vi "Current Loop 9505 (FPGA) - bef combining sample current loops.vi"() -> ()   [LabVIEW 2011]
uses:
  <vilib>/LabVIEW Targets/FPGA/cRIO/cRIO-9505/controls.llb/_nicrio_cRIO-9505_DriveStatus.ctl
  <vilib>/Platform/TimedLoop/XDataNode/timing_clust.ctl
  <vilib>/Platform/TimedLoop/XDataNode/nitl_modes.ctl
  <vilib>/Platform/TimedLoop/XDataNode/wakeup.ctl
  <vilib>/LabVIEW Targets/FPGA/cRIO/cRIO-9505/controls.llb/_nicrio_cRIO-9505_DriveDirection.ctl
  <vilib>/rvi/eio/common/nirviEmuTemplateMethod_errors.vi
  <vilib>/rvi/eio/common/nirviEmuTemplatePropertyGet_noerrors.vi
  <vilib>/Platform/TimedLoop/XDataNode/XDataNode.xnode
  <vilib>/eio/EIONode/EIONode.xnode
  <vilib>/eio/EIOMethodNode/EIOMethodNode.xnode
  <vilib>/eio/EIOPropertyNode/EIOPropertyNode.xnode
  <vilib>/Platform/TimedLoop/XDataNode/XDNodeRunTimeDep.lvlib
  <vilib>/rvi/eio/common/nirviEmuTemplatePropertyGet_errors.vi
  <vilib>/rvi/eio/common/nirviEmuTemplatePropertySet_errors.vi
  <vilib>/rvi/eio/common/nirviEmuTemplatePropertySet_noerrors.vi
panel:
  in  "Trig AI 2":bool
  out "Vsup Present 2":bool
  out "Drive Fault 2":bool
  out "Drive Status 2":T1
  out "Temp Fault 2":bool
  in  "Enable\nDrive 2":bool
  in  "Disable\nDrive 2":bool
  in  "Current PI gains 2":T2={"Proportional Gain"=20, "Integral Gain"=10, "Derivative Gain"=0}
  in  "Current Feedback 2":i16
  in  "Current Limit 2":i16 caption="Setpoint"
  in  "Current Setpoint 2":i16 caption="Setpoint"
  in  "Current Loop\nRate (usec) 2":u32=50
  out "PWM Duty Cycle 2":i16
  in  "Current PI gains":T2={"Proportional Gain"=20, "Integral Gain"=10, "Derivative Gain"=0}
  in  "Current Limit":i16 caption="Setpoint"
  in  "Current Setpoint":i16 caption="Setpoint"
  in  "Current Loop\nRate (usec)":u32=50
  out "Vsup Present":bool
  out "Drive Fault":bool
  out "Drive Status":T1
  out "Temp Fault":bool
  in  "Enable\nDrive":bool
  in  "Disable\nDrive":bool
  in  "Trig AI":bool
  in  "Current Feedback":i16
  out "PWM Duty Cycle":i16
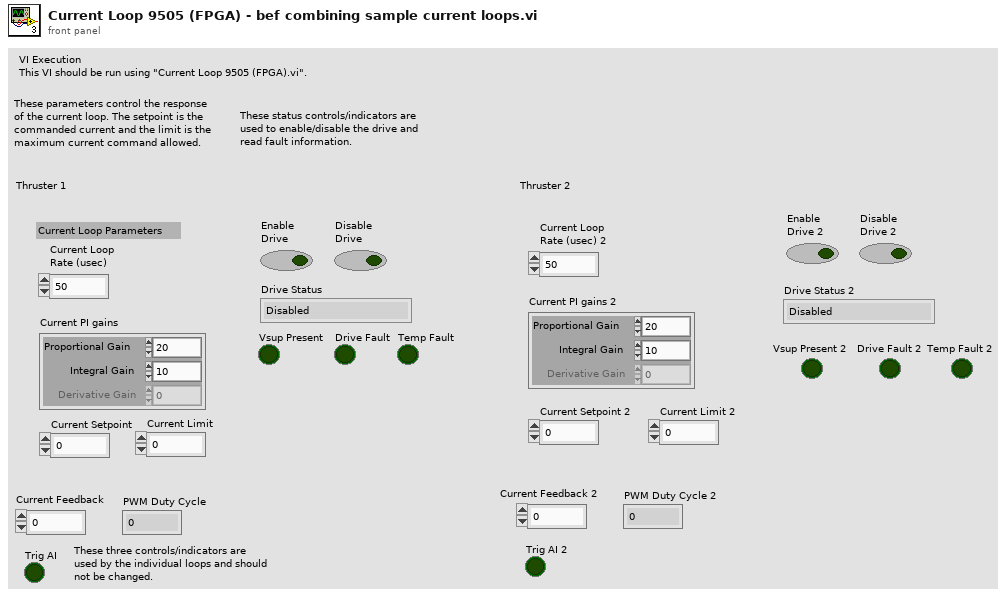
[diagram p1: front panel]
types:
  T1 = typedef "_nicrio_cRIO-9505_DriveStatus.ctl" = enum8{"Enabled", "Disabled", "Disabled by Drive Fault", "Disabled by Temp. Fault", "Disabled by E-Stop", "Unknown"}
  T2 = cluster{"Proportional Gain":i16, "Integral Gain":i16, "Derivative Gain":i16}
  T3 = typedef "XDNodeRunTimeDep.lvlib/timing_clust.ctl" = cluster{"Expected End [f-1]":u64, "Actual End [f-1]":u64, "Finished Late? [f-1]":bool, "Expected End [i-1]":u64, "Actual End [i-1]":u64, "Finished Late? [i-1]":bool, "Expected Start [i]":u64, "Actual Start [i]":u64, "Expected Start [f]":u64, "Actual Start [f]":u64, "Source Name":string, "Structure Name":string, "Period":i64, "Deadline":i64, "Offset":i64, "Start":i64, "Priority":i32, "Timeout":i32, "Mode":T4, "Wakeup Reason":T5, "Error":errorcluster, "Source Type":string, "Secondary Source Type":string, "Global End Time":u64, "Global Start Time":u64, "Frame Duration":u64, "Iteration Duration":u64, "Assigned CPU":i32, "I/O Scan Engine Mode":u32}
  T4 = typedef "XDNodeRunTimeDep.lvlib/nitl_modes.ctl" = enum32{"No Change", "Process missed periods, maintain original phase", "Discard missed periods, maintain original phase", "Process missed periods, ignore original phase", "Discard missed periods, ignore original phase"}
  T5 = typedef "XDNodeRunTimeDep.lvlib/wakeup.ctl" = enum32{"Normal", "Aborted", "Asynchronous wakeup", "Timing source error", "Timed loop error", "Timeout"}
  T6 = typedef "_nicrio_cRIO-9505_DriveDirection.ctl" = enum8{"Clockwise", "Counterclockwise"}
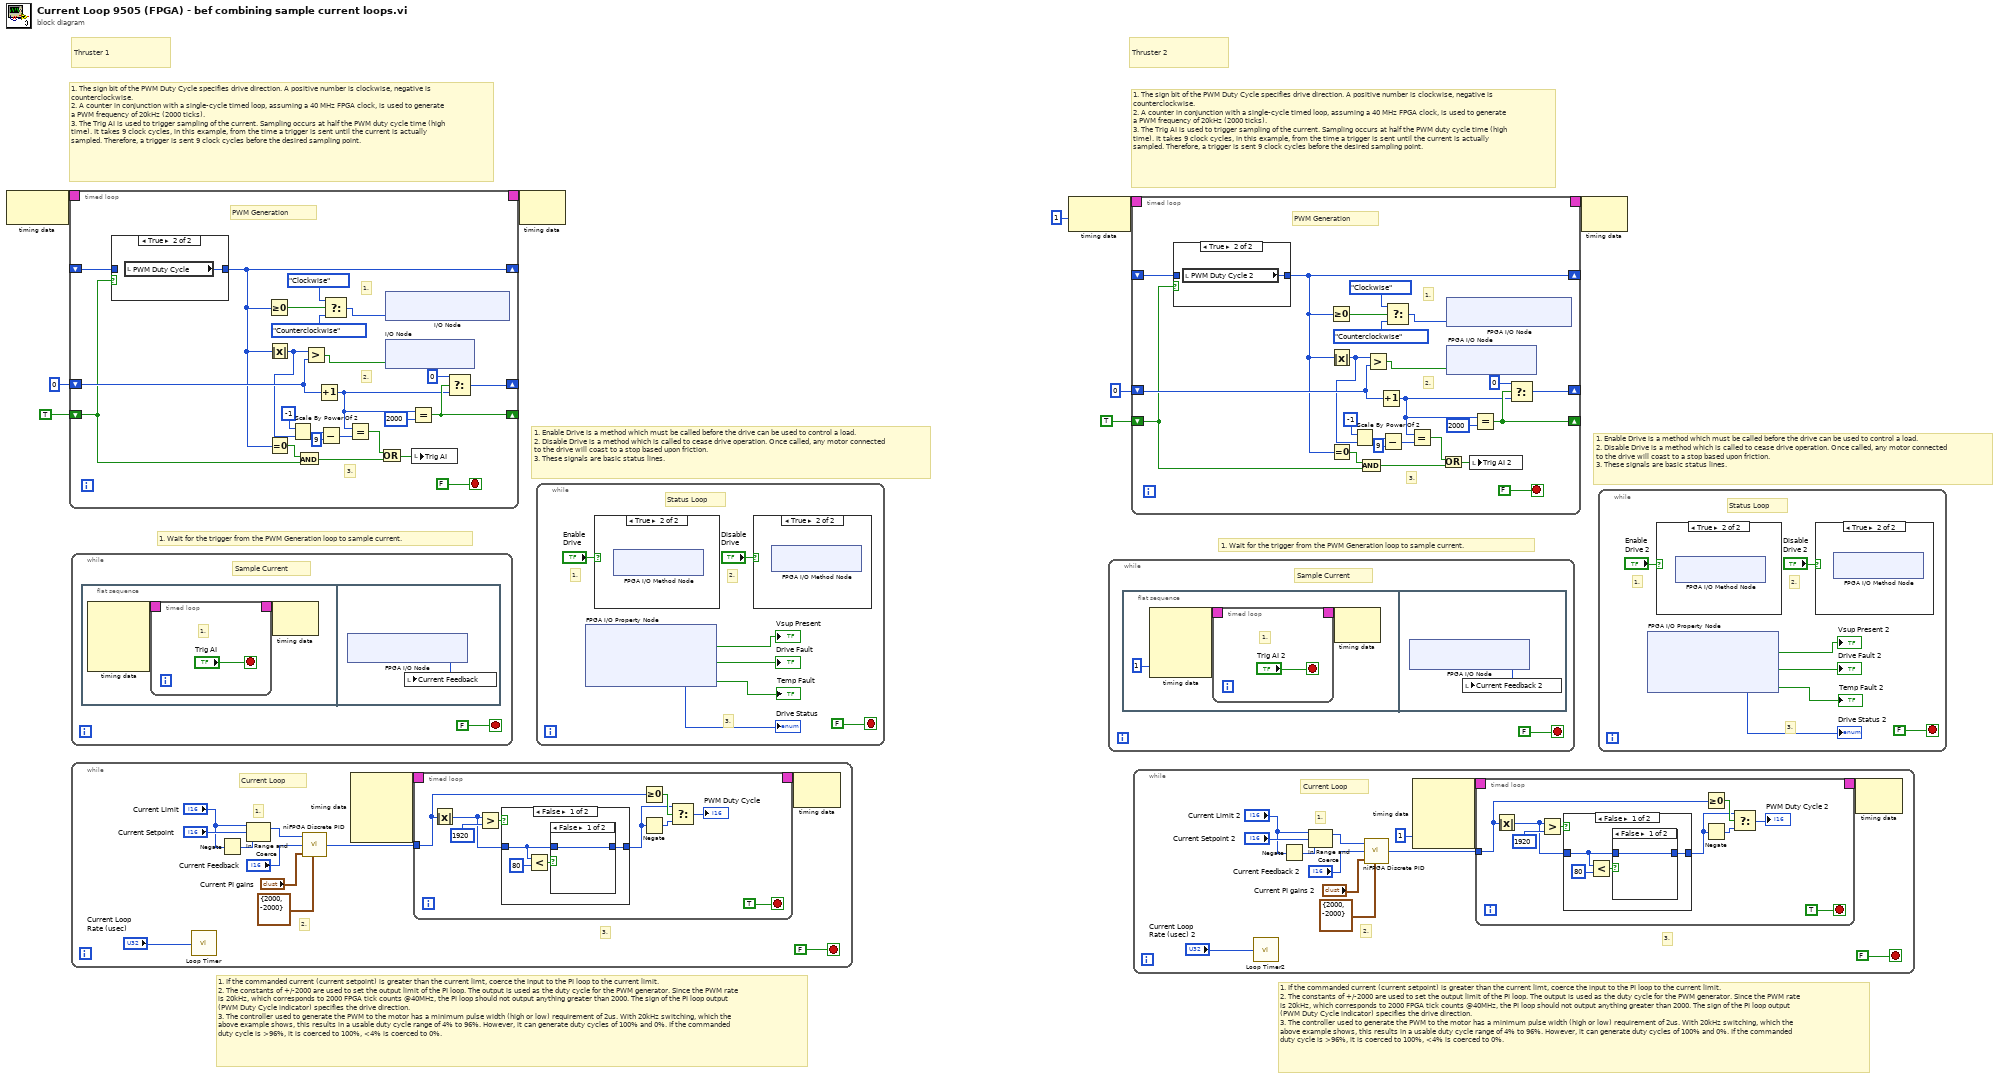
[diagram p0: block diagram]
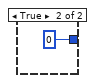
[diagram p5: hidden frame]
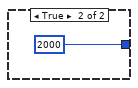
[diagram p6: hidden frame]
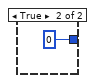
[diagram p10: hidden frame]
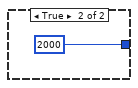
[diagram p11: hidden frame]
diagram:
  # "Thruster 2"
  # "Thruster 1"
  # "1. Enable Drive is a method which must be called before the drive can be used to control a load.\n2. Disable Drive is a method which is called to cease drive operation. Once called, any motor connected to the drive will coast to a stop based upon friction.\n3. These signals are basic status lines."
  # "1. Wait for the trigger from the PWM Generation loop to sample current."
  # "1. The sign bit of the PWM Duty Cycle specifies drive direction. A positive number is clockwise, negative is counterclockwise.\n2. A counter in conjunction with a single-cycle timed loop, assuming a 40 MHz FPGA clock, is used to generate a PWM frequency of 20kHz (2000 ticks).\n3. The Trig AI is used to trigger sampling of the current. Sampling occurs at half the PWM duty cycle time (high time). It takes 9 clock cycles, in this example, from the time a trigger is sent until the current is actually sampled. Therefore, a trigger is sent 9 clock cycles before the desired sampling point."
  # "1. If the commanded current (current setpoint) is greater than the current limt, coerce the input to the PI loop to the current limit.\n2. The constants of +/-2000 are used to set the output limit of the PI loop. The output is used as the duty cycle for the PWM generator. Since the PWM rate is 20kHz, which corresponds to 2000 FPGA tick counts @40MHz, the PI loop should not output anything greater than 2000. The sign of the PI loop output (PWM Duty Cycle indicator) specifies the drive direction.\n3. The controller used to generate the PWM to the motor has a minimum pulse width (high or low) requirement of 2us. With 20kHz switching, which the above example shows, this results in a usable duty cycle range of 4% to 96%. However, it can generate duty cycles of 100% and 0%. If the commanded duty c..."
  # "1. Enable Drive is a method which must be called before the drive can be used to control a load.\n2. Disable Drive is a method which is called to cease drive operation. Once called, any motor connected to the drive will coast to a stop based upon friction.\n3. These signals are basic status lines."
  # "1. Wait for the trigger from the PWM Generation loop to sample current."
  # "1. The sign bit of the PWM Duty Cycle specifies drive direction. A positive number is clockwise, negative is counterclockwise.\n2. A counter in conjunction with a single-cycle timed loop, assuming a 40 MHz FPGA clock, is used to generate a PWM frequency of 20kHz (2000 ticks).\n3. The Trig AI is used to trigger sampling of the current. Sampling occurs at half the PWM duty cycle time (high time). It takes 9 clock cycles, in this example, from the time a trigger is sent until the current is actually sampled. Therefore, a trigger is sent 9 clock cycles before the desired sampling point."
  # "1. If the commanded current (current setpoint) is greater than the current limt, coerce the input to the PI loop to the current limit.\n2. The constants of +/-2000 are used to set the output limit of the PI loop. The output is used as the duty cycle for the PWM generator. Since the PWM rate is 20kHz, which corresponds to 2000 FPGA tick counts @40MHz, the PI loop should not output anything greater than 2000. The sign of the PI loop output (PWM Duty Cycle indicator) specifies the drive direction.\n3. The controller used to generate the PWM to the motor has a minimum pulse width (high or low) requirement of 2us. With 20kHz switching, which the above example shows, this results in a usable duty cycle range of 4% to 96%. However, it can generate duty cycles of 100% and 0%. If the commanded duty c..."
  n1 = node-c288() -> (w9:T3)  [unwired: 1 out]
  n2 = timed-loop {
    timing: w9 -> [_]
    timing-out: [_] -> w8
    shift-right: [w30] -> _
    shift-left: i16 0 -> [w33]
    shift-right: [w29] -> _
    shift-left: TRUE -> [w26]
    shift-right: [w15] -> _
    shift-left: _ -> [w28]
    stop <- FALSE stop-if-true
    # "3."
    # "2."
    # "1."
    # "PWM Generation"
    n3 = case shown="True" w26 {
      tunnel: [w34 w35] -> w15
      tunnel: w28 -> [w34 _]
      frame False {
      }
      frame True {
        n4 = local read "PWM Duty Cycle"() -> (w35:i16)
      }
    }
    n5 = Greater Or Equal To 0?(x=w15) -> (x >= 0?=w22:bool)
    n6 = Absolute Value(x=w15) -> (abs(x)=w13:i16)
    n7 = Equal To 0?(x=w15) -> (x = 0?=w27:bool)
    n8 = Scale By Power Of 2(n=i8 -1, x=w13) -> (x*2^n=w17:i16)
    n9 = And(x=w27, y=w26) -> (x .and. y?=w23:bool)
    n10 = Greater?(x=w13, y=w33) -> (0:w11:bool)
    n11 = Increment(x=w33) -> (x+1=w25:i16)
    n12 = Subtract(x=w17, y=i8 9) -> (x-y=w16:i16)
    n13 = Select(t=_nicrio_cRIO-9505_DriveDirection."Clockwise", s=w22, f=_nicrio_cRIO-9505_DriveDirection."Counterclockwise") -> (s? t:f=w10:T6)
    n14 = Equal?(x=w25, y=w16) -> (x = y?=w24:bool)
    n15 = Or(x=w24, y=w23) -> (x .or. y?=w19:bool)
    n16 = xnode "I/O Node"("Mod2/Drive Direction"=w10) -> ()  [unwired: 1 in, 1 out]
    n17 = xnode "I/O Node"("Mod2/Motor"=w11) -> ()  [unwired: 1 in, 1 out]
    n18 = Equal?(x=w25, y=i16 2000) -> (x = y?=w29:bool)
    n19 = local write "Trig AI"(w19) -> ()
    n20 = Select(t=i16 0, s=w29, f=w25) -> (s? t:f=w30:i16)
  }
  n21 = while {
    stop <- FALSE stop-if-true
    # "Sample Current"
    n22 = flat-sequence {
      frame #0 {
        n23 = node-c288() -> (w40:T3)  [unwired: 4 out]
        n24 = timed-loop {
          timing: w40 -> [_]
          timing-out: [_] -> w39
          stop <- "Trig AI" stop-if-true
          # "1."
        }
        n25 = node-c288(w39) -> ()  [unwired: 1 out]
      }
      frame #1 {
        n26 = xnode "FPGA I/O Node"() -> ("Mod2/Current Sense"=w46:i16)  [unwired: 1 in, 1 out]
        n27 = local write "Current Feedback"(w46) -> ()
      }
    }
  }
  n28 = while {
    stop <- FALSE stop-if-true
    # "3."
    # "2."
    # "1."
    # "Current Loop"
    n29 = call "Loop Timer"("Count(uSec)"="Current Loop\nRate (usec)") -> ()  [unwired: 1 out]
    n30 = Negate(x="Current Limit") -> (-x=w51:i16)
    n31 = In Range and Coerce(upper limit="Current Limit", x="Current Setpoint", lower limit=w51) -> (coerced(x)=w49:i16)  [unwired: 1 out]
    n32 = call <vilib>:"niFPGA Discrete PID.vi"("setpoint"=w49, "process variable"="Current Feedback", "PID gains (x 2^8)"="Current PI gains", "output range"=cluster{"output high":i16, "output low":i16} {"output high"=2000, "output low"=-2000}) -> ("output"=w55:i16)  [unwired: 1 in, 4 out]
    n33 = node-c288() -> (w54:T3)  [unwired: 4 out]
    n34 = timed-loop {
      timing: w54 -> [_]
      timing-out: [_] -> w53
      tunnel: w55 -> [w61]
      stop <- TRUE stop-if-true
      n35 = Absolute Value(x=w61) -> (abs(x)=w62:i16)
      n36 = Greater?(x=w62, y=i16 1920) -> (0:w64:bool)
      n37 = case shown="False" w64 {
        tunnel: [w70 i16 2000] -> w63
        tunnel: w62 -> [w68 _]
        frame False {
          n38 = Less?(x=w68, y=i16 80) -> (x < y?=w69:bool)
          n39 = case shown="False" w69 {
            tunnel: [w72 i16 0] -> w70
            tunnel: w68 -> [w72 _]
            frame False {
            }
            frame True {
            }
          }
        }
        frame True {
        }
      }
      n40 = Greater Or Equal To 0?(x=w61) -> (x >= 0?=w67:bool)
      n41 = Negate(x=w63) -> (-x=w66:i16)
      n42 = Select(t=w63, s=w67, f=w66) -> (s? t:f=→"PWM Duty Cycle":i16)
    }
    n43 = node-c288(w53) -> ()  [unwired: 1 out]
  }
  n44 = node-c288(w8) -> ()  [unwired: 1 out]
  n45 = while {
    stop <- FALSE stop-if-true
    # "3."
    # "2."
    # "1."
    # "Status Loop"
    n46 = xnode "FPGA I/O Property Node"() -> ("Vsup Present"=→"Vsup Present":bool, "Drive Fault"=→"Drive Fault":bool, "Drive Status"=→"Drive Status":T1, "Over Temperature Fault"=→"Temp Fault":bool)  [unwired: 1 in, 1 out]
    n47 = case shown="True" "Enable\nDrive" {
      frame False {
      }
      frame True {
        n48 = xnode "FPGA I/O Method Node"() -> ()  [unwired: 1 in, 1 out]
      }
    }
    n49 = case shown="True" "Disable\nDrive" {
      frame False {
      }
      frame True {
        n50 = xnode "FPGA I/O Method Node"() -> ()  [unwired: 1 in, 1 out]
      }
    }
  }
  n51 = node-c288(1) -> (w5:T3)
  n52 = while {
    stop <- FALSE stop-if-true
    # "Sample Current"
    n53 = flat-sequence {
      frame #0 {
        n54 = node-c288(1) -> (w89:T3)  [unwired: 3 out]
        n55 = timed-loop {
          timing: w89 -> [_]
          timing-out: [_] -> w88
          stop <- "Trig AI 2" stop-if-true
          # "1."
        }
        n56 = node-c288(w88) -> ()  [unwired: 1 out]
      }
      frame #1 {
        n57 = xnode "FPGA I/O Node"() -> ("Mod4/Current Sense"=w97:i16)  [unwired: 1 in, 1 out]
        n58 = local write "Current Feedback 2"(w97) -> ()
      }
    }
  }
  n59 = timed-loop {
    timing: w5 -> [_]
    timing-out: [_] -> w4
    shift-right: [w118] -> _
    shift-left: i16 0 -> [w121]
    shift-right: [w117] -> _
    shift-left: TRUE -> [w114]
    shift-right: [w103] -> _
    shift-left: _ -> [w116]
    stop <- FALSE stop-if-true
    # "3."
    # "2."
    # "1."
    # "PWM Generation"
    n60 = case shown="True" w114 {
      tunnel: [w122 w123] -> w103
      tunnel: w116 -> [w122 _]
      frame False {
      }
      frame True {
        n61 = local read "PWM Duty Cycle 2"() -> (w123:i16)
      }
    }
    n62 = Greater Or Equal To 0?(x=w103) -> (x >= 0?=w110:bool)
    n63 = Absolute Value(x=w103) -> (abs(x)=w101:i16)
    n64 = Equal To 0?(x=w103) -> (x = 0?=w115:bool)
    n65 = Scale By Power Of 2(n=i8 -1, x=w101) -> (x*2^n=w105:i16)
    n66 = And(x=w115, y=w114) -> (x .and. y?=w111:bool)
    n67 = Greater?(x=w101, y=w121) -> (0:w99:bool)
    n68 = Increment(x=w121) -> (x+1=w113:i16)
    n69 = Subtract(x=w105, y=i8 9) -> (x-y=w104:i16)
    n70 = Select(t=_nicrio_cRIO-9505_DriveDirection."Clockwise", s=w110, f=_nicrio_cRIO-9505_DriveDirection."Counterclockwise") -> (s? t:f=w98:T6)
    n71 = Equal?(x=w113, y=w104) -> (x = y?=w112:bool)
    n72 = Or(x=w112, y=w111) -> (x .or. y?=w107:bool)
    n73 = xnode "FPGA I/O Node"("Mod4/Drive Direction"=w98) -> ()  [unwired: 1 in, 1 out]
    n74 = xnode "FPGA I/O Node"("Mod4/Motor"=w99) -> ()  [unwired: 1 in, 1 out]
    n75 = local write "Trig AI 2"(w107) -> ()
    n76 = Equal?(x=w113, y=i16 2000) -> (x = y?=w117:bool)
    n77 = Select(t=i16 0, s=w117, f=w113) -> (s? t:f=w118:i16)
  }
  n78 = while {
    stop <- FALSE stop-if-true
    # "3."
    # "2."
    # "1."
    # "Current Loop"
    n79 = call "Loop Timer2"("Count(uSec)"="Current Loop\nRate (usec) 2") -> ()  [unwired: 1 out]
    n80 = Negate(x="Current Limit 2") -> (-x=w131:i16)
    n81 = In Range and Coerce(upper limit="Current Limit 2", x="Current Setpoint 2", lower limit=w131) -> (coerced(x)=w129:i16)  [unwired: 1 out]
    n82 = call <vilib>:"niFPGA Discrete PID.vi"("setpoint"=w129, "process variable"="Current Feedback 2", "PID gains (x 2^8)"="Current PI gains 2", "output range"=cluster{"output high":i16, "output low":i16} {"output high"=2000, "output low"=-2000}) -> ("output"=w135:i16)  [unwired: 1 in, 4 out]
    n83 = node-c288(1) -> (w134:T3)  [unwired: 3 out]
    n84 = timed-loop {
      timing: w134 -> [_]
      timing-out: [_] -> w133
      tunnel: w135 -> [w141]
      stop <- TRUE stop-if-true
      n85 = Absolute Value(x=w141) -> (abs(x)=w142:i16)
      n86 = Greater?(x=w142, y=i16 1920) -> (0:w144:bool)
      n87 = case shown="False" w144 {
        tunnel: [w150 i16 2000] -> w143
        tunnel: w142 -> [w148 _]
        frame False {
          n88 = Less?(x=w148, y=i16 80) -> (x < y?=w149:bool)
          n89 = case shown="False" w149 {
            tunnel: [w152 i16 0] -> w150
            tunnel: w148 -> [w152 _]
            frame False {
            }
            frame True {
            }
          }
        }
        frame True {
        }
      }
      n90 = Greater Or Equal To 0?(x=w141) -> (x >= 0?=w147:bool)
      n91 = Negate(x=w143) -> (-x=w146:i16)
      n92 = Select(t=w143, s=w147, f=w146) -> (s? t:f=→"PWM Duty Cycle 2":i16)
    }
    n93 = node-c288(w133) -> ()  [unwired: 1 out]
  }
  n94 = node-c288(w4) -> ()  [unwired: 1 out]
  n95 = while {
    stop <- FALSE stop-if-true
    # "3."
    # "2."
    # "1."
    # "Status Loop"
    n96 = xnode "FPGA I/O Property Node"() -> ("Vsup Present"=→"Vsup Present 2":bool, "Drive Fault"=→"Drive Fault 2":bool, "Drive Status"=→"Drive Status 2":T1, "Over Temperature Fault"=→"Temp Fault 2":bool)  [unwired: 1 in, 1 out]
    n97 = case shown="True" "Enable\nDrive 2" {
      frame False {
      }
      frame True {
        n98 = xnode "FPGA I/O Method Node"() -> ()  [unwired: 1 in, 1 out]
      }
    }
    n99 = case shown="True" "Disable\nDrive 2" {
      frame False {
      }
      frame True {
        n100 = xnode "FPGA I/O Method Node"() -> ()  [unwired: 1 in, 1 out]
      }
    }
  }
